vi "-Retrieve_Process_ID_And_Key.vi"(8 "error in (no error)":errorcluster, 11 "Postgres Connector In":refnum<class "Postgres Connector.lvclass">) -> (0 "error out":errorcluster, 3 "Postgres Connector Out":refnum<class "Postgres Connector.lvclass">)   [LabVIEW 2020, in "Postgres Connector.lvclass"]
doc: "This VI is used to retrieve the Process ID and the Secret Key of the connection so it will be possible to cancel a query if desired"
uses:
  Postgres Connector.lvclass
  Postgres Connector.lvclass/Postgres Connector.ctl
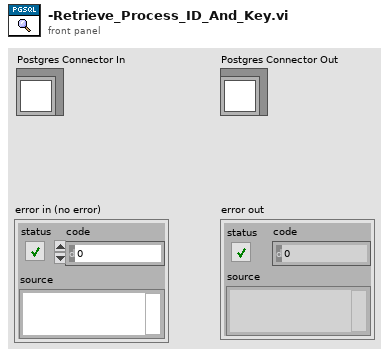
[diagram p1: front panel]
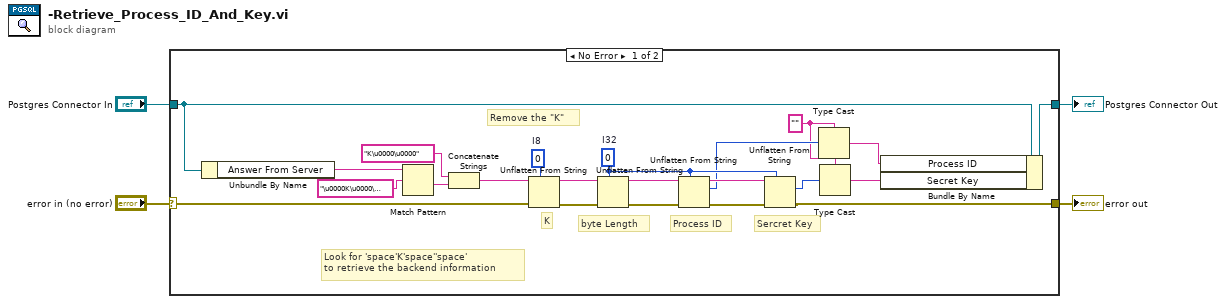
[diagram p0: block diagram]
diagram:
  n1 = case shown="No Error" "error in (no error)" {
    selector: "error in (no error)" -> [w16 w28]
    tunnel: "Postgres Connector In" -> [w11 w27]
    tunnel: [w12 w28] -> w1
    tunnel: [w10 w27] -> w3
    frame No Error {
      w8 = ""
      w19 = i8 0  # I8
      w17 = 0  # I32
      # "Sercret Key"
      # "Process ID"
      # "byte Length"
      # "K"
      # "Look for 'space'K'space''space'\nto retrieve the backend information"
      # "Remove the \"K\""
      n2 = Unbundle By Name(w11) -> ("Answer From Server"=w18:string)
      n3 = Match Pattern(string=w18, regular expression="\u0000K\u0000\u0000") -> (after substring=w22:string)  [unwired: 1 in, 3 out]
      n4 = Concatenate Strings("K\u0000\u0000", w22) -> (w25:string)
      n5 = Unflatten From String(type=w19, binary string=w25, error in (no error)=w16) -> (rest of the binary string=w26:string, error out=w15:errorcluster)  [unwired: 2 in, 1 out]
      n6 = Unflatten From String(type=w17, binary string=w26, error in (no error)=w15) -> (rest of the binary string=w23:string, error out=w14:errorcluster)  [unwired: 2 in, 1 out]
      n7 = Unflatten From String(type=w17, binary string=w23, error in (no error)=w14) -> (rest of the binary string=w24:string, value=w9:i32, error out=w13:errorcluster)  [unwired: 2 in]
      n8 = Unflatten From String(type=w17, binary string=w24, error in (no error)=w13) -> (value=w5:i32, error out=w12:errorcluster)  [unwired: 2 in, 1 out]
      n9 = Type Cast(type=w8, x=w9) -> (*(type *) &x=w7:string)
      n10 = Type Cast(type=w8, x=w5) -> (*(type *) &x=w6:string)
      n11 = Bundle By Name(cluster=w11, "Process ID"=w7, "Secret Key"=w6) -> (w10:refnum<class "Postgres Connector.lvclass">)
    }
    frame Error {
    }
  }
  "Postgres Connector Out" <- w3
  "error out" <- w1
